vi "Biclusters.vi"(8 "error in (no error)":errorcluster caption="entrée d'erreur (pas d'erreur)", 11 "make_biclusters":T2={"n_rows"=300, "n_cols"=300, "n_clusters"=5, "noise"=5.0, "minval"=10, "maxval"=100, "shuffle"=TRUE, "random_state"=-1, "Returns"="X"} {"random_state" min=-1; "n_clusters" min=1; "n_cols" min=1; "n_rows" min=1}) -> (0 "error out":errorcluster, 3 "Data":T1)   [LabVIEW 2020]
doc: "Generate an array with constant block diagonal structure for biclustering.\n\n\nParameters :\n\n- shape : iterable (n_rows, n_cols)\nThe shape of the result.\n\n- n_clusters : integer\nThe number of biclusters.\n\n- noise : float, optional (default=0.0)\nThe standard deviation of the gaussian noise.\n\n- minval : int, optional (default=10)\nMinimum value of a bicluster.\n\n- maxval : int, optional (default=100)\nMaximum value of a bicluster.\n\n- shuffle : boolean, optional (default=True)\nShuffle the samples.\n\n- random_state : int, RandomState instance, default=None=-1\nDetermines random number generation for dataset creation. Pass an int for reproducible output across multiple function calls. See Glossary.\n\nReturns : \n\n- X : array of shape shape\nThe generated array.\n\n- rows : array of shape (n_clusters, X.shape[0],)\nThe indicators for cluster membership of each row.\n\n- cols : array of shape (n_clusters, X.shape[1],)\nThe indicators for cluster membership of each column."
uses:
  Biclusters.lvclass
panel:
  out "Biclusters.lvclass":refnum<class "Biclusters.lvclass">
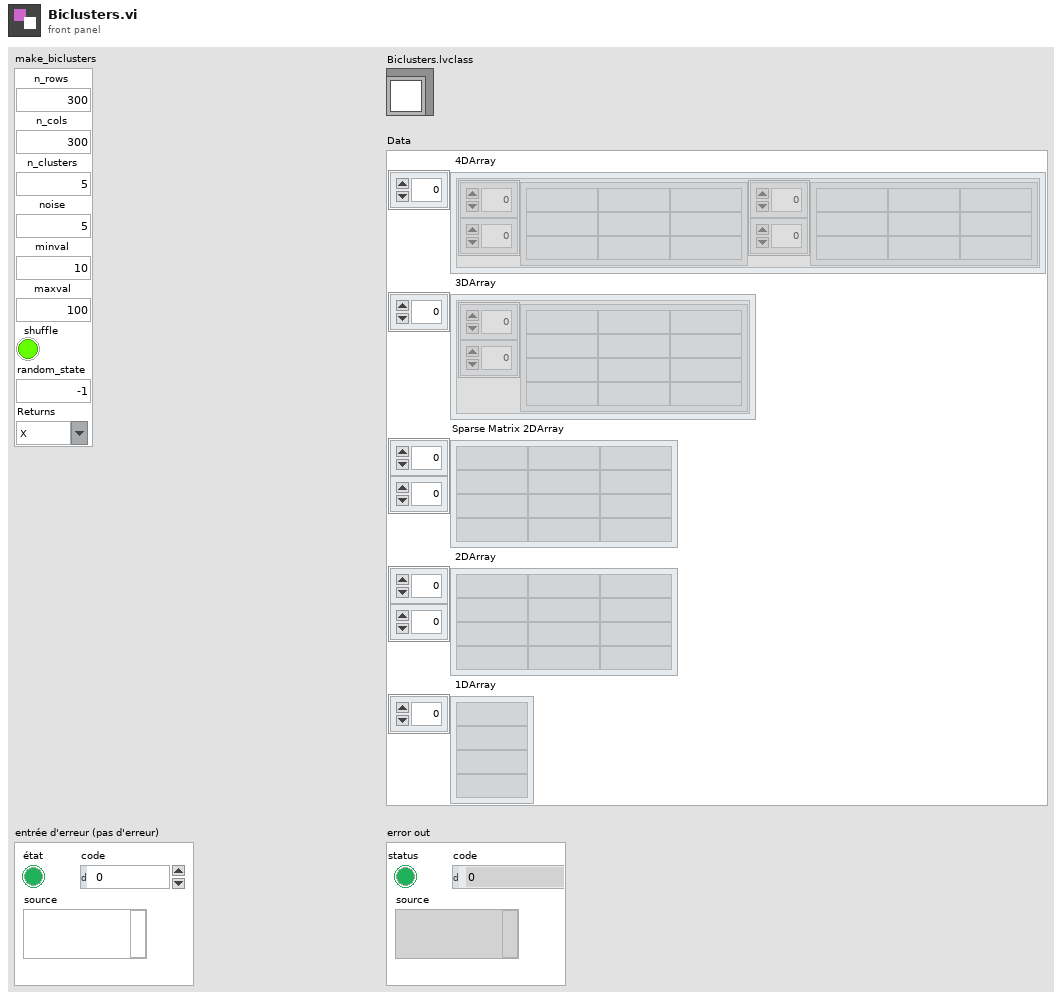
[diagram p1: front panel]
types:
  T1 = cluster{" 4DArray":cluster{"1":string[][], "2":string[][]}[], " 3DArray":cluster{"Tableau":string[][]}[], "Sparse Matrix 2DArray":string[][], " 2DArray":string[][], " 1DArray":string[]}
  T2 = cluster{"n_rows":u32, "n_cols":u32, "n_clusters":u32, "noise":dbl, "minval":i32, "maxval":i32, "shuffle":bool, "random_state":i32, "Returns":string}
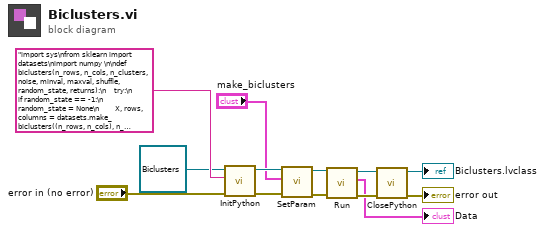
[diagram p0: block diagram]
diagram:
  n1 = call-dynamic "InitPython.vi"("error in (no error)"="error in (no error)", "Python Instruction"="import sys\nfrom sklearn import datasets\nimport numpy \n\ndef biclusters(n_rows, n_cols, n_clusters, noise, minval, maxval, shuffle, random_state, returns):\n    try:\n        if random_state == -1:\n            random_state = None\n        X, rows, columns = datasets.make_biclusters((n_rows, n_cols), n_clusters, noise, minval, maxval, shuffle, random_state)\n        if returns == 'X':\n            dataX = X.tolist()\n            return str(dataX)\n        elif returns == 'rows' :\n            data_rows = rows.tolist()\n            return str(data_rows)\n        else:\n            data_columns = columns.tolist()\n            return str(data_columns)\n    except:\n        erreur = sys.exc_info()\n        typerr = u\"%s\" % (erreur[0])\n        typerr = typerr[typerr.find(\"'\")+1:typerr.rfind(\"'\")]\n        msgerr = u\"%s\" % (erreur[1])\n        message = str('/!\\\\ {0} : {1}'. format(typerr,msgerr))\n        return message", "Scikit-learn en entrée"=refnum<class "Biclusters.lvclass"> refnum ("Biclusters.lvclass")) -> ("error out"=w10:errorcluster, "Scikit-learn en sortie"=w11:refnum<class "Biclusters.lvclass">)  [unwired: 7 in]
  n2 = call-dynamic "SetParam.vi"("error in (no error)"=w10, "make_biclusters"="make_biclusters", "Biclusters.lvclass"=w11) -> ("error out"=w6:errorcluster, "Biclusters.lvclass"=w7:refnum<class "Biclusters.lvclass">)  [unwired: 7 in]
  n3 = call-dynamic "Run.vi"("error in (no error)"=w6, "Biclusters.lvclass"=w7) -> ("error out"=w4:errorcluster, "Data"=→"Data":T1, "Biclusters.lvclass"=w5:refnum<class "Biclusters.lvclass">)  [unwired: 7 in]
  n4 = call-dynamic "ClosePython.vi"("error in (no error)"=w4, "Scikit-learn en entrée"=w5) -> ("error out"=→"error out":errorcluster, "Scikit-learn en sortie"=→"Biclusters.lvclass":refnum<class "Biclusters.lvclass">)  [unwired: 8 in]
